vi "UE9 PWM and Counter Loop.vi"(8 "error in":errorcluster, 9 "PWM Duty Cycle [%]":dbl=50.0 format="%.1f", 10 "PWM Frequency [Hz]":dbl=1000.0 format="%.1f") -> (0 "error out":errorcluster, 2 "Actual Frequency":dbl format="%.1f")   [LabVIEW 2021]
panel:
  out "Total Counts":u32
  in  "stop":bool
  out "Current Counter0 Read":u32
  in  "FirstFound":bool=TRUE
  in  "Address":string="1"
  in  "ConnectionType":u16(ring) items=["LJ_ctUSB", "LJ_ctETHERNET"]
  out "PWM Timer Value":u16
  out "TimerClockDivisor":u8
  out "TimerClockBase":string
  out "Error Message":string
  # "Demonstrates 1 channel of 8-bit PWM output and 1 hardware counter.  Short FIO0 (PWM output)\nto FIO1 (hardware counter).  Runs in a loop where we can change frequency and duty cycle while\nrunning.  Keeps track of total number of pulses, which turns out to be a little tricky.\n\nTimer clock base and timer clock divisor, are chosen to get as close as possible to the desired PWM frequency.\nFor 660<=f<=187500, system clock is used for timer clock.\nFor f<660, fixed 750kHz timer clock is used for timer clock."
  # "187500 Hz max, 11.4 Hz min"
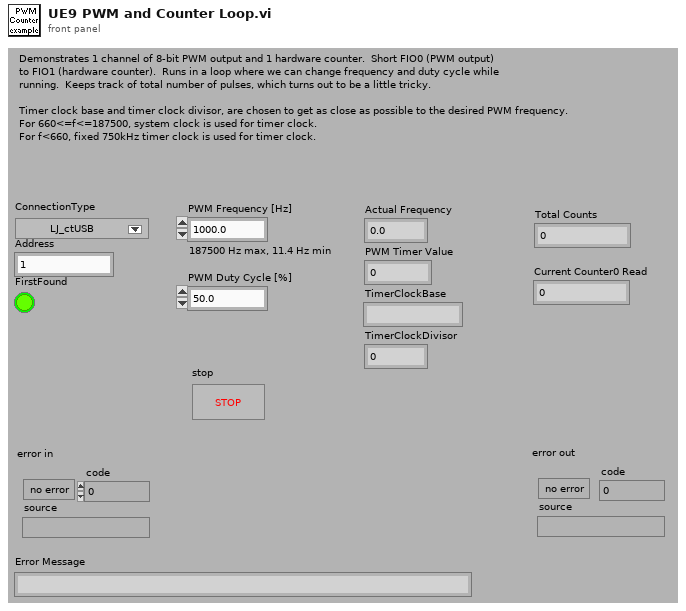
[diagram p1: front panel]
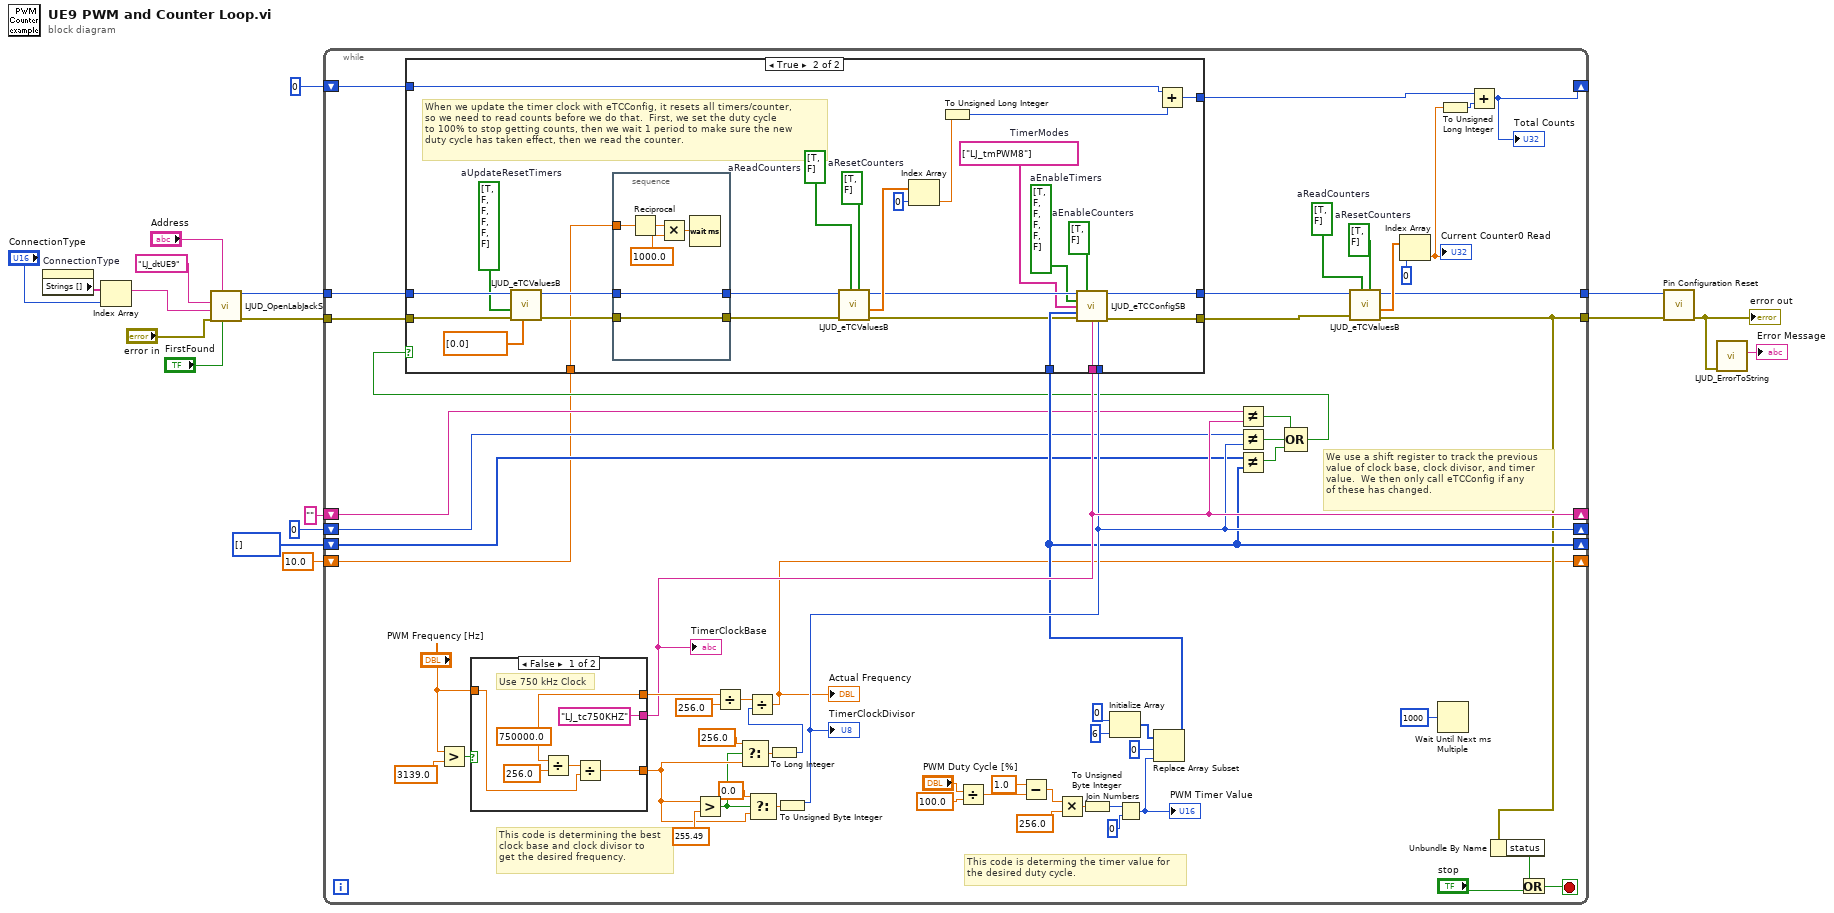
[diagram p0: block diagram]
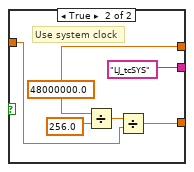
[diagram p3: hidden frame]
diagram:
  n1 = property on="ConnectionType" class="Ring (strict)"() -> ("Strings []"=w13:string[])  [unwired: 2 in, 2 out]
  n2 = Index Array(array=w13, index="ConnectionType") -> (element=w11:string)
  n3 = call "LJUD_OpenLabJackS.vi"("FirstFound"="FirstFound", "Address"="Address", "error in"="error in", "ConnectionType"=w11, "DeviceType"="LJ_dtUE9") -> ("error out"=w9:errorcluster, "Handle"=w10:i32)  [unwired: 4 in, 1 out]
  n4 = while {
    shift-left: 10.0 -> [w19]
    shift-right: [w20] -> _
    shift-left: u32 0 -> [w24]
    shift-right: [w27] -> _
    shift-left: u16[] [] -> [w38]
    shift-right: [w39] -> _
    shift-left: u8 0 -> [w21]
    shift-right: [w40] -> _
    shift-left: "" -> [w22]
    shift-right: [w41] -> _
    tunnel: [w31] -> w7
    tunnel: [w45] -> w8
    tunnel: w9 -> [w46]
    tunnel: w10 -> [w47]
    stop <- w30 stop-if-true
    w28 = bool[] [TRUE, FALSE]  # aResetCounters
    w29 = bool[] [TRUE, FALSE]  # aReadCounters
    # "We use a shift register to track the previous\nvalue of clock base, clock divisor, and timer\nvalue.  We then only call eTCConfig if any\nof these has changed."
    # "This code is determing the timer value for\nthe desired duty cycle."
    # "This code is determining the best\nclock base and clock divisor to\nget the desired frequency."
    n5 = Greater?(x="PWM Frequency [Hz]", y=3139.0) -> (0:w61:bool)
    n6 = case shown="False" w61 {
      tunnel: "PWM Frequency [Hz]" -> [w117 w123]
      tunnel: [w116 w122] -> w50
      tunnel: [w115 w121] -> w72
      tunnel: ["LJ_tc750KHZ" "LJ_tcSYS"] -> w41
      frame False {
        w115 = 750000.0 ("x")
        # "Use 750 kHz Clock"
        n7 = Divide(x=w115, y=256.0) -> (x/y=w119:dbl)
        n8 = Divide(x=w119, y=w117) -> (x/y=w116:dbl)
      }
      frame True {
        w121 = 48000000.0 ("x")
        # "Use system clock"
        n9 = Divide(x=w121, y=256.0) -> (x/y=w125:dbl)
        n10 = Divide(x=w125, y=w123) -> (x/y=w122:dbl)
      }
    }
    "TimerClockBase" <- w41
    n11 = Greater?(x=w50, y=255.49) -> (0:w49:bool)
    n12 = Divide(x=w72, y=256.0) -> (x/y=w74:dbl)
    n13 = Select(t=256.0, s=w49, f=w50) -> (s? t:f=w52:dbl)
    n14 = Select(t=0.0, s=w49, f=w50) -> (s? t:f=w75:dbl)
    n15 = To Long Integer(number=w52) -> (32bit integer=w48:i32)
    n16 = Divide(x=w74, y=w48) -> (x/y=w20:dbl)
    "Actual Frequency" <- w20
    n17 = To Unsigned Byte Integer(number=w75) -> (unsigned 8bit integer=w40:u8)
    "TimerClockDivisor" <- w40
    n18 = Divide(x="PWM Duty Cycle [%]", y=100.0) -> (x/y=w68:dbl)
    n19 = Subtract(x=1.0, y=w68) -> (x-y=w66:dbl)
    n20 = Multiply(x=w66, y=256.0) -> (x*y=w63:dbl)
    n21 = To Unsigned Byte Integer(number=w63) -> (unsigned 8bit integer=w65:u8)
    n22 = Initialize Array(u16 0 ("PWM Timer Value"), 6 ("Dimension Size")) -> (w55:u16[])
    n23 = Join Numbers(hi=w65, lo=u8 0) -> ((hi.lo)=w54:u16)
    "PWM Timer Value" <- w54
    n24 = Replace Array Subset(array=w55, new element=w54, index=0 ("Index")) -> (w39:u16[])
    n25 = Not Equal?(x=w22, y=w41) -> (x != y?=w37:bool)
    n26 = Not Equal?(x=w21, y=w40) -> (x != y?=w36:bool)
    n27 = Not Equal?(x=w38, y=w39) -> (x != y?=w35:bool)
    n28 = Compound Arithmetic op=OR(w37, w36, w35) -> (w34:bool)
    n29 = case shown="True" w34 {
      tunnel: w47 -> [w80 w89]
      tunnel: w46 -> [w79 w88]
      tunnel: [w79 w107] -> w44
      tunnel: [w80 w106] -> w43
      tunnel: w39 -> [_ w105]
      tunnel: w40 -> [_ w104]
      tunnel: w41 -> [_ w103]
      tunnel: w24 -> [w78 w95]
      tunnel: [w78 w96] -> w23
      tunnel: w19 -> [_ w81]
      frame False {
      }
      frame True {
        w87 = bool[] [TRUE, FALSE, FALSE, FALSE, FALSE, FALSE]  # aUpdateResetTimers
        w101 = bool[] [TRUE, FALSE]  # aReadCounters
        w102 = bool[] [TRUE, FALSE]  # aResetCounters
        w90 = string[] ["LJ_tmPWM8"]  # TimerModes
        w91 = bool[] [TRUE, FALSE, FALSE, FALSE, FALSE, FALSE]  # aEnableTimers
        w92 = bool[] [TRUE, FALSE]  # aEnableCounters
        # "When we update the timer clock with eTCConfig, it resets all timers/counter,\nso we need to read counts before we do that.  First, we set the duty cycle\nto 100% to stop getting counts, then we wait 1 period to make sure the new\nduty cycle has taken effect, then we read the counter."
        n30 = call "LJUD_eTCValuesB.vi"("aTimerValues Write"=dbl[] [0.0], "error in"=w88, "aUpdateResetTimers"=w87, "Handle In"=w89) -> ("error out"=w85:errorcluster, "Handle Out"=w84:i32)  [unwired: 4 in, 2 out]
        n31 = stacked-sequence {
          tunnel: w85 -> [w112]
          tunnel: w84 -> [w113]
          tunnel: [w113] -> w83
          tunnel: [w112] -> w82
          tunnel: w81 -> [w108]
          frame #0 {
            n32 = Reciprocal(x=w108) -> (1/x=w111:dbl)
            n33 = Multiply(x=w111, y=1000.0) -> (x*y=w109:dbl)
            n34 = Wait (ms)(milliseconds to wait=w109) -> ()  [unwired: 1 out]
          }
        }
        n35 = call "LJUD_eTCValuesB.vi"("aResetCounters"=w102, "aReadCounters"=w101, "error in"=w82, "Handle In"=w83) -> ("error out"=w97:errorcluster, "aCounterValues"=w99:dbl[], "Handle Out"=w98:i32)  [unwired: 4 in, 1 out]
        n36 = Index Array(array=w99, index=0 ("Index")) -> (element=w93:dbl)
        n37 = To Unsigned Long Integer(number=w93) -> (unsigned 32bit integer=w94:u32)
        n38 = call "LJUD_eTCConfigSB.vi"("Handle In"=w98, "aEnableCounters"=w92, "aEnableTimers"=w91, "aTimerModes"=w90, "aTimerValues"=w105, "error in"=w97, "TimerClockBase"=w103, "TimerClockDivisor"=w104) -> ("Handle Out"=w106:i32, "error out"=w107:errorcluster)  [unwired: 6 in]
        n39 = Add(x=w95, y=w94) -> (x+y=w96:u32)
      }
    }
    n40 = call "LJUD_eTCValuesB.vi"("aResetCounters"=w28, "aReadCounters"=w29, "error in"=w44, "Handle In"=w43) -> ("error out"=w31:errorcluster, "aCounterValues"=w59:dbl[], "Handle Out"=w45:i32)  [unwired: 4 in, 1 out]
    n41 = Index Array(array=w59, index=0 ("Index")) -> (element=w25:dbl)
    "Current Counter0 Read" <- w25
    n42 = Wait Until Next ms Multiple(millisecond multiple=u32 1000) -> ()  [unwired: 1 out]
    n43 = To Unsigned Long Integer(number=w25) -> (unsigned 32bit integer=w26:u32)
    n44 = Add(x=w23, y=w26) -> (x+y=w27:u32)
    "Total Counts" <- w27
    n45 = Unbundle By Name(w31) -> ("status"=w33:bool)
    n46 = Or(x=w33, y="stop") -> (x .or. y?=w30:bool)
  }
  n47 = call "Pin Configuration Reset.vi"("error in"=w7, "Handle In"=w8) -> ("error out"=w6:errorcluster)  [unwired: 8 in, 1 out]
  "error out" <- w6
  n48 = call "LJUD_ErrorToString.vi"("error in"=w6) -> ("String"=→"Error Message":string)  [unwired: 10 in]
